vi "Turn off pump.vi"(9 "Boolean":bool, 10 "Announce":dbl, 11 "Numeric":dbl) -> (3 "In Range?":bool)   [LabVIEW 2023]
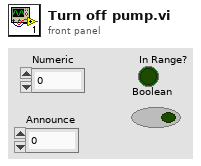
[diagram p1: front panel]
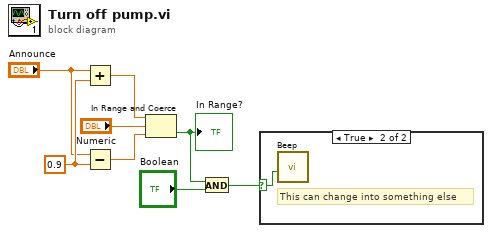
[diagram p0: block diagram]
diagram:
  w8 = 0.9
  n1 = Add(x="Announce", y=w8) -> (x+y=w6:dbl)
  n2 = Subtract(x="Announce", y=w8) -> (x-y=w5:dbl)
  n3 = In Range and Coerce(upper limit=w6, x="Numeric", lower limit=w5) -> (In Range?=w2:bool)  [unwired: 1 out]
  "In Range?" <- w2
  n4 = And(x=w2, y="Boolean") -> (x .and. y?=w1:bool)
  n5 = case shown="True" w1 {
    selector: w1 -> [_ w9]
    frame False {
    }
    frame True {
      # "This can change into something else"
      n6 = call <vilib>:"Beep.vi"("use system alert? (T)"=w9) -> ()  [unwired: 11 in]
    }
  }
